vi "Test OO.vi"() -> ()   [LabVIEW 2020]
uses:
  Objects/Saving Function/Saving OO/Saving OO.lvclass
panel:
  in  "Array":string[][](array[string])
  out "Data":string[][](array[string])
  in  "Saving OO in":refnum<class "Saving OO.lvclass">
  in  "Path":path
  in  "error in (no error)":errorcluster
  out "Saving OO out":refnum<class "Saving OO.lvclass">
  out "error out":errorcluster
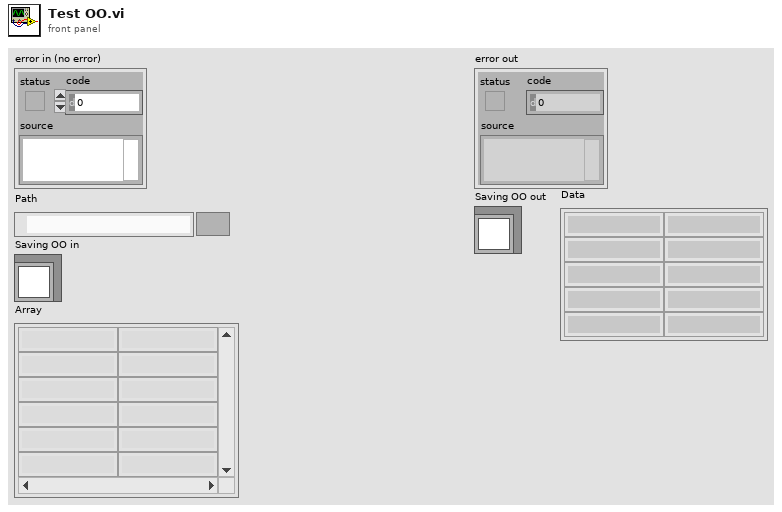
[diagram p1: front panel]
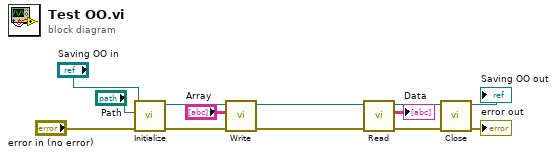
[diagram p0: block diagram]
diagram:
  n1 = call-dynamic "Initialize.vi"("error in (no error)"="error in (no error)", "Path"="Path", "Saving OO in"="Saving OO in") -> ("error out"=w12:errorcluster, "Saving OO out"=w13:refnum<class "Saving OO.lvclass">)  [unwired: 7 in]
  n2 = call-dynamic "Write.vi"("error in (no error)"=w12, "Array"="Array", "Saving OO in"=w13) -> ("error out"=w10:errorcluster, "Saving OO out"=w11:refnum<class "Saving OO.lvclass">)  [unwired: 7 in]
  n3 = call-dynamic "Read.vi"("error in (no error)"=w10, "Saving OO in"=w11) -> ("error out"=w8:errorcluster, "Data"=→"Data":string[][], "Saving OO out"=w9:refnum<class "Saving OO.lvclass">)  [unwired: 7 in]
  n4 = call-dynamic "Close.vi"("error in (no error)"=w8, "Saving OO in"=w9) -> ("error out"=→"error out":errorcluster, "Saving OO out"=→"Saving OO out":refnum<class "Saving OO.lvclass">)  [unwired: 8 in]
